vi "mouse down action.vi"(8 "engine":refnum<data-value>, 10 "CtlRef":refnum<vi>, 11 "module editor reference":refnum<data-value>) -> (0 "error out":errorcluster)   [LabVIEW 2013]
uses:
  <vilib>/NI/Tag Bus Data Framework/control module/configuration/control module configuration.lvclass
  <vilib>/NI/Tag Bus/tag/tag descriptor.lvclass
  <vilib>/NI/Configuration Framework/serializable configuration/NISE_CEF_serializable configuration.lvclass
  <vilib>/NI/Module Execution Interface/Engine Configuration/engine configuration.lvclass
  <vilib>/NI/Tag Bus Data Framework/Configuration Editor/Classes/Engine Parent/Engine Parent Editor Node.lvclass
  <vilib>/NI/Tag Bus Data Framework/control module/editor node/control module editor.lvclass
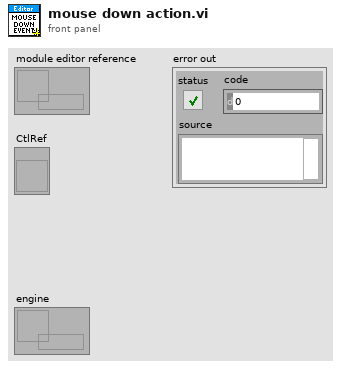
[diagram p1: front panel]
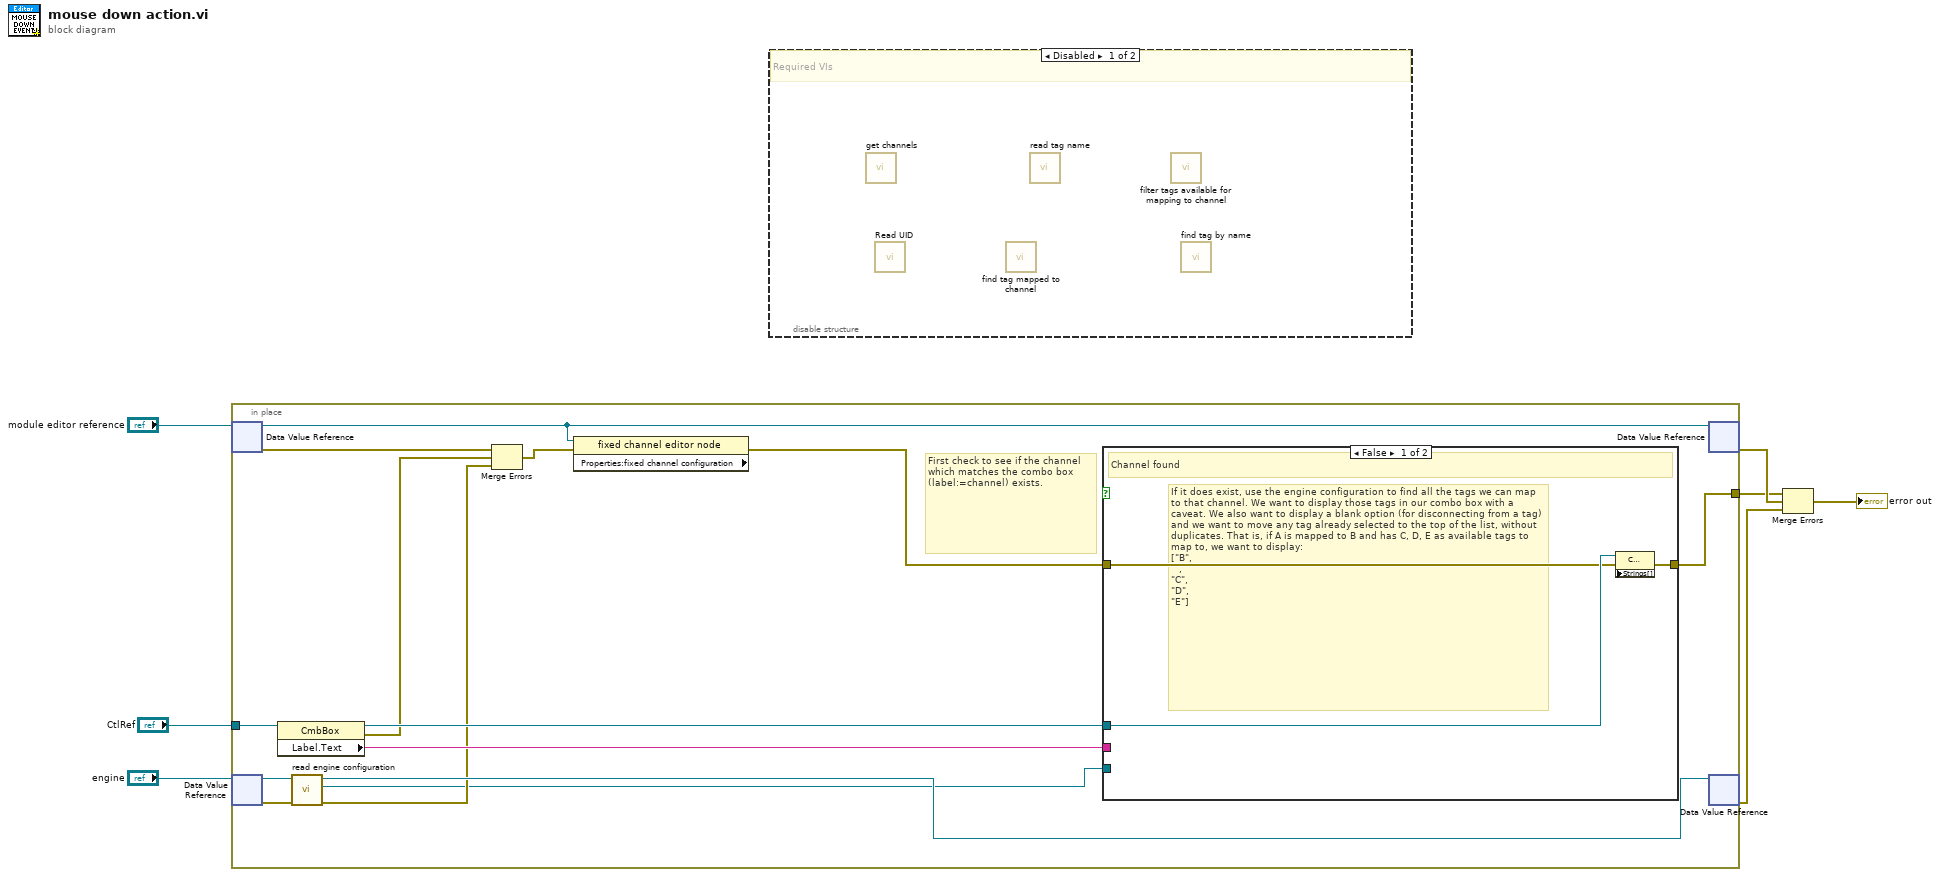
[diagram p0: block diagram]
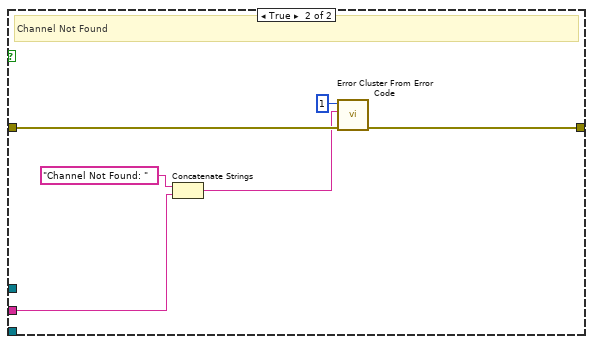
[diagram p3: hidden frame]
diagram:
  n1 = in-place {
    in-place-border: [w20] -> w2
    in-place-border: "CtlRef" -> [w18]
    # "First check to see if the channel which matches the combo box (label:=channel) exists."
    n2 = in-place-dvr #1("module editor reference") -> (w16:refnum<class "control module editor.lvclass">, w21:errorcluster)
    n3 = in-place-dvr #2("engine") -> (w13:refnum<class "Engine Parent Editor Node.lvclass">, w11:errorcluster)
    n4 = property class="CmbBox"(reference=w18) -> (reference out=w15:refnum<vi>, error out=w10:errorcluster, "Label.Text"=w14:string)  [unwired: 1 in]
    n5 = call <vilib>:"read engine configuration.vi"("error in"=w11, "Engine Parent Editor Node in"=w13) -> ("error out"=w9:errorcluster, "engine configuration"=w8:refnum<class "engine configuration.lvclass">, "Engine Parent Editor Node out"=w12:refnum<class "Engine Parent Editor Node.lvclass">)  [unwired: 7 in]
    n6 = Merge Errors(w21, w10, w9) -> (w17:errorcluster)
    n7 = property class="fixed channel editor node" props=["Properties:fixed channel configuration"](reference=w16, error in=w17) -> (error out=w19:errorcluster)  [unwired: 2 out]
    n8 = case shown="False" {
      selector: _ -> [_ _]
      tunnel: [w23 w29] -> w20
      tunnel: w19 -> [w22 w28]
      tunnel: w15 -> [w24 _]
      tunnel: w14 -> [_ w26]
      tunnel: w8 -> [_ _]
      frame False {
        # "If it does exist, use the engine configuration to find all the tags we can map to that channel. We want to display those tags in our combo box with a caveat. We also want to display a blank option (for disconnecting from a tag) and we want to move any tag already selected to the top of the list, without duplicates. That is, if A is mapped to B and has C, D, E as available tags to map to, we want to display:\n[\"B\",\n\"\",\n\"C\",\n\"D\",\n\"E\"]"
        # "Channel found"
        n9 = property class="CmbBox" props=["Strings[]"](reference=w24, error in=w22) -> (error out=w23:errorcluster)  [unwired: 1 in, 1 out]
      }
      frame True {
        # "Channel Not Found"
        n10 = Concatenate Strings("Channel Not Found: " ("string"), w26) -> (w25:string)
        n11 = call <vilib>:"Error Cluster From Error Code.vi"("error in (no error)"=w28, "error message (\"\")"=w25, "error code (0)"=1) -> ("error out"=w29:errorcluster)  [unwired: 6 in]
      }
    }
    n12 = in-place-dvr #1(w16) -> (w3:errorcluster)  [unwired: 1 out]
    n13 = in-place-dvr #2(w12) -> (w6:errorcluster)  [unwired: 1 out]
  }
  n14 = disable-structure shown="Disabled" {
    frame Disabled {
      # "Required VIs"
      n15 = call-dynamic "get channels.vi"() -> ()  [unwired: 10 in, 2 out]
      n16 = call <vilib>:"Read UID.vi"() -> ()  [unwired: 9 in, 3 out]
      n17 = call <vilib>:"find tag mapped to channel.vi"() -> ()  [unwired: 9 in, 3 out]
      n18 = call <vilib>:"read tag name.vi"() -> ()  [unwired: 9 in, 3 out]
      n19 = call <vilib>:"filter tags available for mapping to channel.vi"() -> ()  [unwired: 10 in, 2 out]
      n20 = call <vilib>:"find tag by name.vi"() -> ()  [unwired: 11 in, 1 out]
    }
    frame Enabled {
    }
  }
  n21 = Merge Errors(w2, w3, w6) -> (→"error out":errorcluster)
